vi "Get TCPIP Message.vi"(8 "error in (no error)":errorcluster, 11 "Channel Manager in":refnum<class "Channel Manager.lvclass">) -> (0 "error out":errorcluster, 3 "Channel Manager out":refnum<class "Channel Manager.lvclass">)   [LabVIEW 2018, in "Channel Manager.lvclass"]
uses:
  Channel Manager.lvclass
  Channel Manager.lvclass/Channel Manager.ctl
  Channel/Channel.lvclass
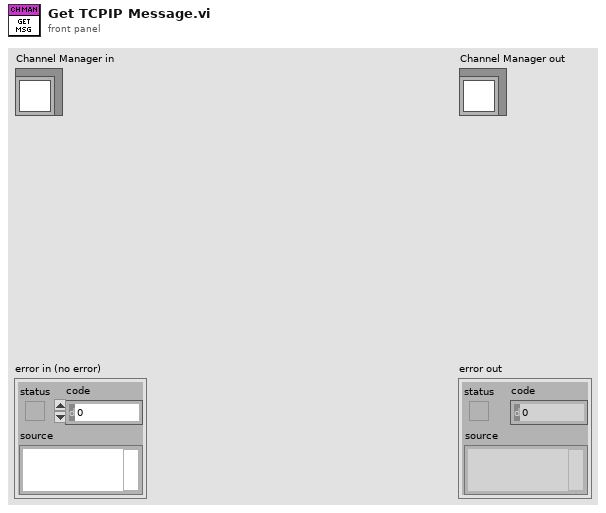
[diagram p1: front panel]
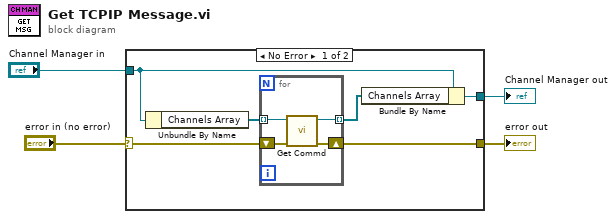
[diagram p0: block diagram]
diagram:
  n1 = case shown="No Error" "error in (no error)" {
    selector: "error in (no error)" -> [w5 w16]
    tunnel: [w6 w16] -> w3
    tunnel: [w8 w15] -> w1
    tunnel: "Channel Manager in" -> [w9 w15]
    frame No Error {
      n2 = Unbundle By Name(w9) -> ("Channels Array"=w10:refnum<class "Channel.lvclass">[])
      n3 = for {
        tunnel: w10 -> [w12] mode=indexing
        shift-right: [w13] -> w6
        shift-left: w5 -> [w14]
        tunnel: [w11] -> w7 mode=indexing
        n4 = call "Get Commd.vi"("error in (no error)"=w14, "Channel in"=w12) -> ("error out"=w13:errorcluster, "Channel out"=w11:refnum<class "Channel.lvclass">)  [unwired: 8 in]
      }
      n5 = Bundle By Name(cluster=w9, "Channels Array"=w7) -> (w8:refnum<class "Channel Manager.lvclass">)
    }
    frame Error {
    }
  }
  "error out" <- w3
  "Channel Manager out" <- w1
